vi "zad1.vi"() -> ()   [LabVIEW 2017]
panel:
  in  "stop":bool
  in  "?":bool
  in  "?":bool
  in  "?":bool
  in  "?":bool
  out "XY Graph":cluster{"Y":dbl[], "Y":dbl[]}[](graph)
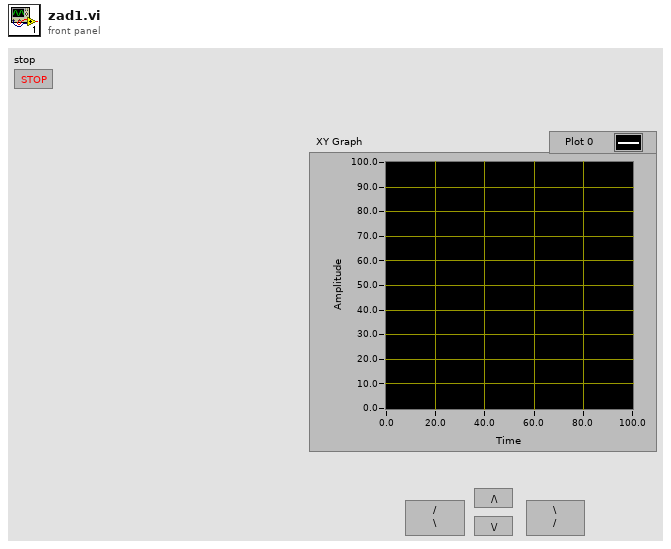
[diagram p1: front panel]
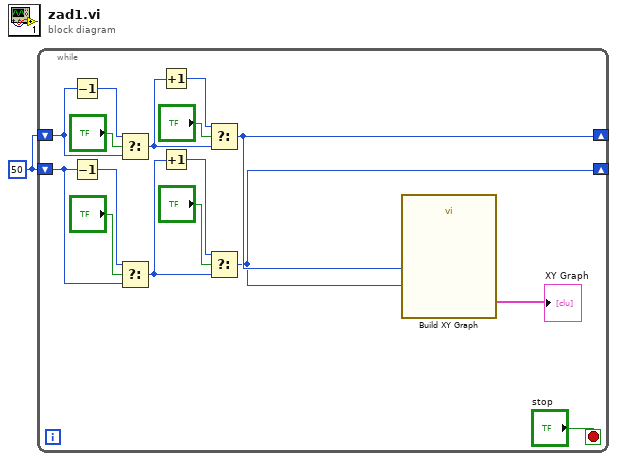
[diagram p0: block diagram]
diagram:
  w1 = 50
  n1 = while {
    shift-right: [w11] -> _
    shift-left: w1 -> [w15]
    shift-right: [w4] -> _
    shift-left: w1 -> [w9]
    stop <- "stop" stop-if-true
    n2 = Decrement(x=w15) -> (x-1=w16:i32)
    n3 = Decrement(x=w9) -> (x-1=w8:i32)
    n4 = Select(t=w16, s="?", f=w15) -> (s? t:f=w12:i32)
    n5 = Select(t=w8, s="?", f=w9) -> (s? t:f=w5:i32)
    n6 = Increment(x=w12) -> (x+1=w13:i32)
    n7 = Increment(x=w5) -> (x+1=w6:i32)
    n8 = Select(t=w13, s="?", f=w12) -> (s? t:f=w11:i32)
    n9 = Select(t=w6, s="?", f=w5) -> (s? t:f=w4:i32)
    n10 = call "Build XY Graph"("Y Input"=w4, "X Input"=w11) -> ("XY Graph"=→"XY Graph":cluster{"X":dbl[], "Y":dbl[]}[])  [unwired: 8 in, 1 out]
  }
